vi "Canread_jetson_L.vi"(7 "Param IN":T1, 8 "배열":T2(array[cluster])) -> (1 "Param Out":T1)   [LabVIEW 2019]
uses:
  6fe196f8-990b-4365-833a-5f23432b79ab.vi
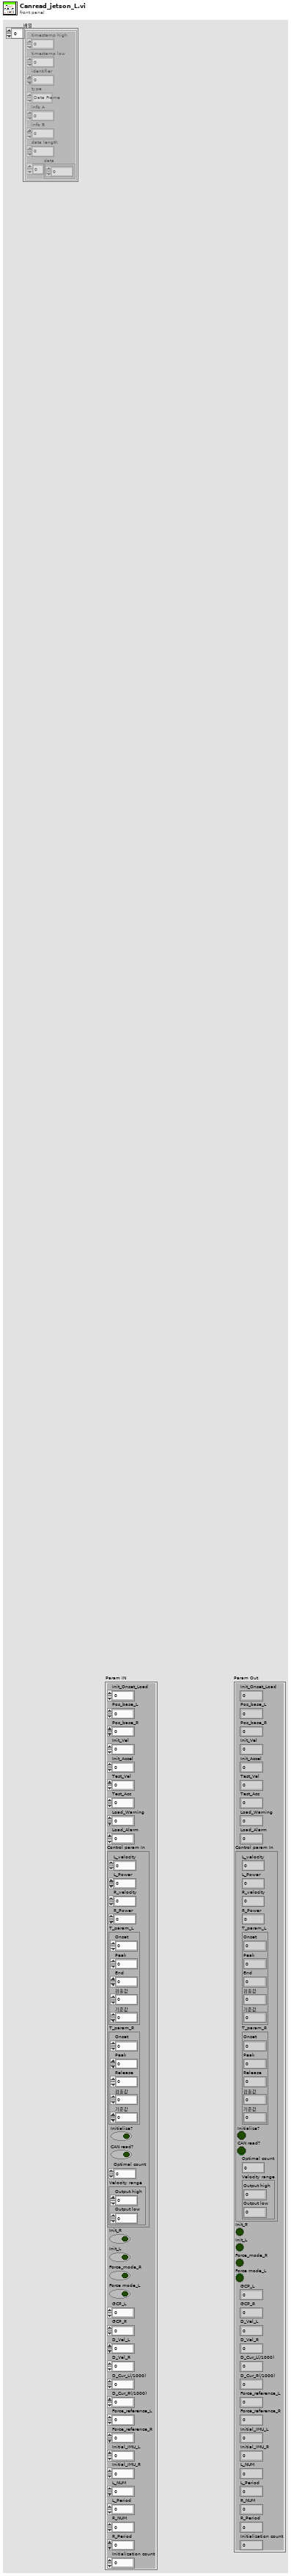
[diagram p1: front panel]
types:
  T1 = cluster{"Init_Onset_Load":sgl, "Pos_base_L":sgl, "Pos_base_R":sgl, "Init_Vel":i32, "Init_Accel":u32, "Test_Vel":i32, "Test_Acc":u32, "Load_Warning":sgl, "Load_Alarm":sgl, "Control param In":cluster{"L_velocity":u32, "L_Power":sgl, "R_velocity":u32, "R_Power":sgl, "T_param_L":cluster{"Onset":sgl, "Peak":sgl, "End":sgl, "검출값":sgl, "기준값":sgl}, "T_param_R":cluster{"Onset":sgl, "Peak":sgl, "Release":sgl, "검출값":sgl, "기준값":sgl}, "Initialize?":bool, "CAN read?":bool, "Optimal count":i32, "Velocity range":cluster{"Output high":dbl, "Output low":dbl}}, "Init_R":bool, "Init_L":bool, "Force_mode_R":bool, "Force mode_L":bool, "GCP_L":sgl, "GCP_R":sgl, "D_Vel_L":sgl, "D_Vel_R":sgl, "D_Cur_L(/1000)":sgl, "D_Cur_R(/1000)":sgl, "Force_reference_L":sgl, "Force_reference_R":sgl, "Initial_IMU_L":sgl, "Initial_IMU_R":sgl, "L_NUM":u32, "L_Period":i16, "R_NUM":u32, "R_Period":i16, "Initialization count":i32}
  T2 = cluster{"timestamp high":u32, "timestamp low":u32, "identifier":u32, "type":enum8{"Data Frame", "Remote Frame", "(reserved)", "(reserved) ", "(reserved)  ", "(reserved)   ", "Bus Error", "Transceiver Fault"}, "info A":u8, "info B":u8, "data length":u8, "data":u8[]}[]
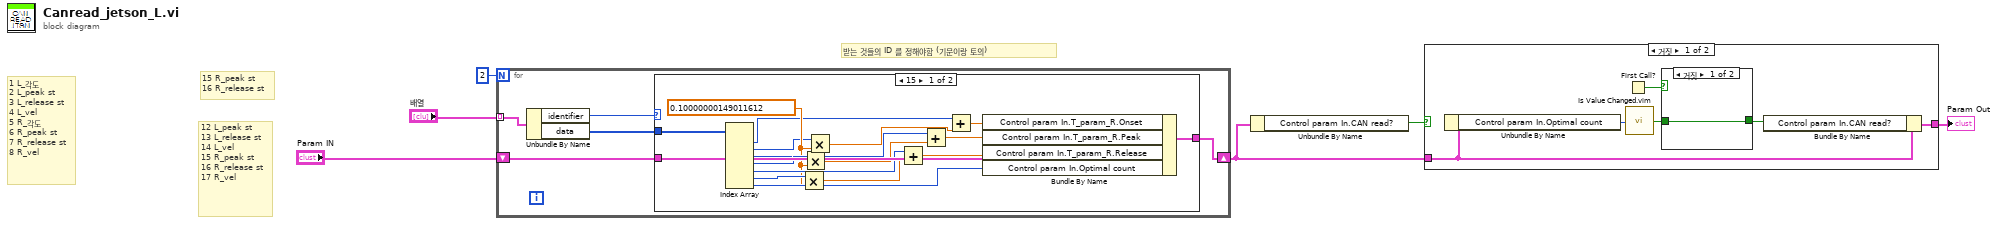
[diagram p0: block diagram]
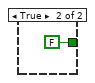
[diagram p2: hidden frame]
diagram:
  # "15 R_peak st\n16 R_release st"
  # "12 L_peak st\n13 L_release st\n14 L_vel\n15 R_peak st\n16 R_release st\n17 R_vel"
  # "받는 것들의 ID 를 정해야함 (기문이랑 토의)"
  # "1 L_각도\n2 L_peak st\n3 L_release st\n4 L_vel\n5 R_각도\n6 R_peak st\n7 R_release st\n8 R_vel"
  n1 = for {
    N: 2 -> [_]
    tunnel: "배열" -> [w11] mode=indexing
    shift-right: [w9] -> w4
    shift-left: "Param IN" -> [w8]
    n2 = Unbundle By Name(w11) -> ("identifier"=w10:u32, "data"=w7:u8[])
    n3 = case shown="15" w10 {
      tunnel: [w27 w29] -> w9
      tunnel: w8 -> [w28 w29]
      tunnel: w7 -> [w24 _]
      frame 15 {
        w16 = sgl 0.1
        n4 = Index Array(array=w24) -> (element #1=w13:u8, element #2=w14:u8, element #3=w18:u8, element #4=w19:u8, element #5=w20:u8, element #6=w22:u8, element #7=w23:u8)  [unwired: 7 in]
        n5 = Multiply(x=w22, y=w16) -> (x*y=w21:sgl)
        n6 = Multiply(x=w19, y=w16) -> (x*y=w17:sgl)
        n7 = Multiply(x=w14, y=w16) -> (x*y=w15:sgl)
        n8 = Add(x=w20, y=w21) -> (x+y=w12:sgl)
        n9 = Add(x=w18, y=w17) -> (x+y=w25:sgl)
        n10 = Add(x=w13, y=w15) -> (x+y=w26:sgl)
        n11 = Bundle By Name(cluster=w28, "Control param In.T_param_R.Onset"=w26, "Control param In.T_param_R.Peak"=w25, "Control param In.T_param_R.Release"=w12, "Control param In.Optimal count"=w23) -> (w27:T1)
      }
      frame 18, Default {
      }
    }
  }
  n12 = Unbundle By Name(w4) -> ("Control param In.CAN read?"=w3:bool)
  n13 = case shown="거짓" w3 {
    tunnel: w4 -> [w34 w37]
    tunnel: [w33 w37] -> w1
    frame False {
      n14 = Unbundle By Name(w34) -> ("Control param In.Optimal count"=w31:i32)
      n15 = First Call?() -> (First Call?: T/F=w32:bool)
      n16 = call "Is Value Changed.vim"("value"=w31) -> ("changed or first call?"=w30:bool)
      n17 = case shown="거짓" w32 {
        tunnel: [w35 FALSE ("changed or first call?")] -> _
        tunnel: w30 -> [w35 _]
        frame False {
        }
        frame True {
        }
      }
      n18 = Bundle By Name(cluster=w34, "Control param In.CAN read?"=w30) -> (w33:T1)
    }
    frame True {
    }
  }
  "Param Out" <- w1
